vi "Create.vi"(8 "error in (no error)":errorcluster) -> (0 "error out":errorcluster, 3 "Current Value Table out":refnum<class "Current Value Table.lvclass">)   [LabVIEW 2024, in "Current Value Table.lvlib" / "Current Value Table.lvclass"]
uses:
  Current Value Table.lvclass
  iCVT_Item/iCVT_Item.lvclass
  Current Value Table.lvclass/Current Value Table.ctl
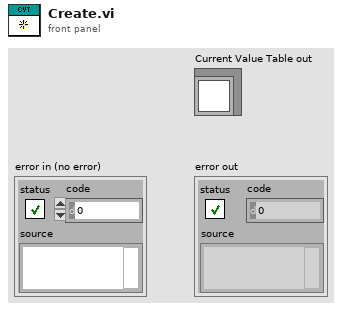
[diagram p1: front panel]
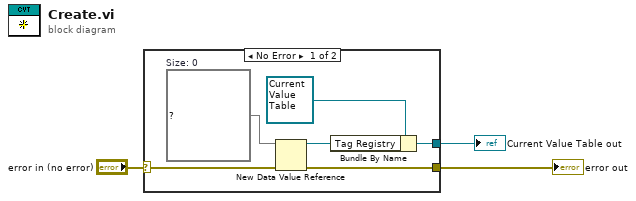
[diagram p0: block diagram]
diagram:
  n1 = case shown="No Error" "error in (no error)" {
    selector: "error in (no error)" -> [w6 w10]
    tunnel: [w5 w10] -> w2
    tunnel: [w7 _] -> w1
    frame No Error {
      w9 = map{string, refnum<class "iCVT_Item.lvclass">} {}  # Size: 0
      n2 = New Data Value Reference(data value=w9, error in=w6) -> (data value reference=w8:refnum<data-value>, error out=w5:errorcluster)
      n3 = Bundle By Name(cluster=refnum<class "Current Value Table.lvclass"> refnum ("Current Value Table.lvlib:Current Value Table.lvclass"), "Tag Registry"=w8) -> (w7:refnum<class "Current Value Table.lvclass">)
    }
    frame Error {
    }
  }
  "error out" <- w2
  "Current Value Table out" <- w1
